vi "Current Min Read Array.vi"(8 "error in":errorcluster, 11 "Power Supply In":refnum<class "Power Supply.lvclass">) -> (0 "error out":errorcluster, 1 "Changed or First Call?":bool, 2 "Current Max SP Limit":dbl[](array[numeric]), 3 "Power Supply Out":refnum<class "Power Supply.lvclass">)   [LabVIEW 2023, in "Power Supply.lvclass"]
uses:
  Power Supply.lvclass
  Power Supply.lvclass/Power Supply.ctl
  Low Level Capabilities/Current/Current Limit/Current Limit.lvclass
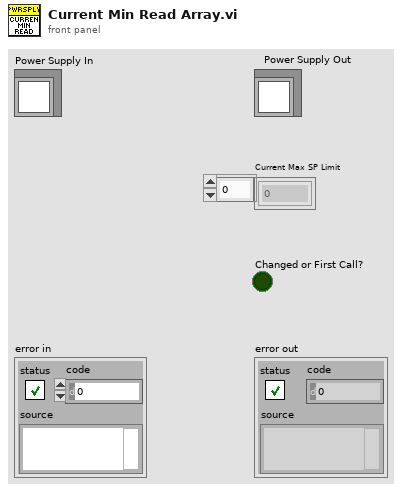
[diagram p1: front panel]
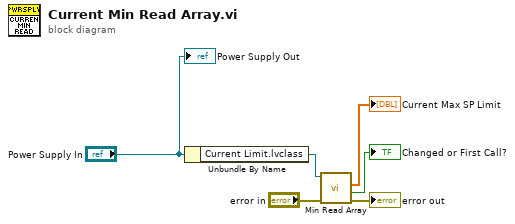
[diagram p0: block diagram]
diagram:
  n1 = Unbundle By Name("Power Supply In") -> ("Current Limit.lvclass"=w1:refnum<class "Current Limit.lvclass">)
  n2 = call-dynamic "Min Read Array.vi"("error in"="error in", "Min Current Limit in"=w1) -> ("error out"=→"error out":errorcluster, "Changed or First Call?"=→"Changed or First Call?":bool, "Current Min SP"=→"Current Max SP Limit":dbl[])  [unwired: 6 in, 1 out]
  "Power Supply Out" <- "Power Supply In"
